vi "CreateProjectsForEachLibrary.vi"() -> ()   [LabVIEW 2019, in "DepsWatchToolsMenu.lvlib"]
uses:
  DepsWatchToolsMenu.lvlib
  vi.lib/DepsWatch/DepsWatch.lvlib
  <userlib>/_OpenG.lib/file/file.llb/Append Path to Root if Relative - Scalar__ogtk.vi
  <userlib>/_OpenG.lib/file/file.llb/Compare Two Paths - Scalar__ogtk.vi
panel:
  out "Projects Created":path[](array[path])
  out "error out":errorcluster
  in  "Build Specs Folder Path":path=path "C:/sw-deps-monitor/Source/BuildSpecs"
  in  "error in (no error)":errorcluster
  in  "Source Folder Path":path=path "C:/sw-deps-monitor/Source"
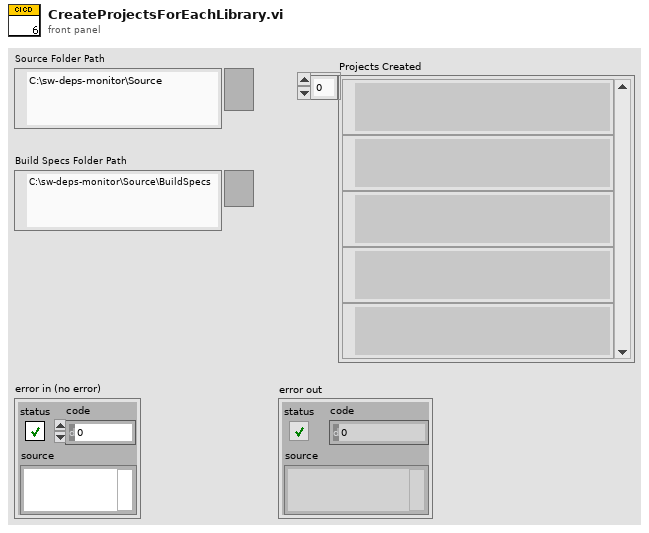
[diagram p1: front panel]
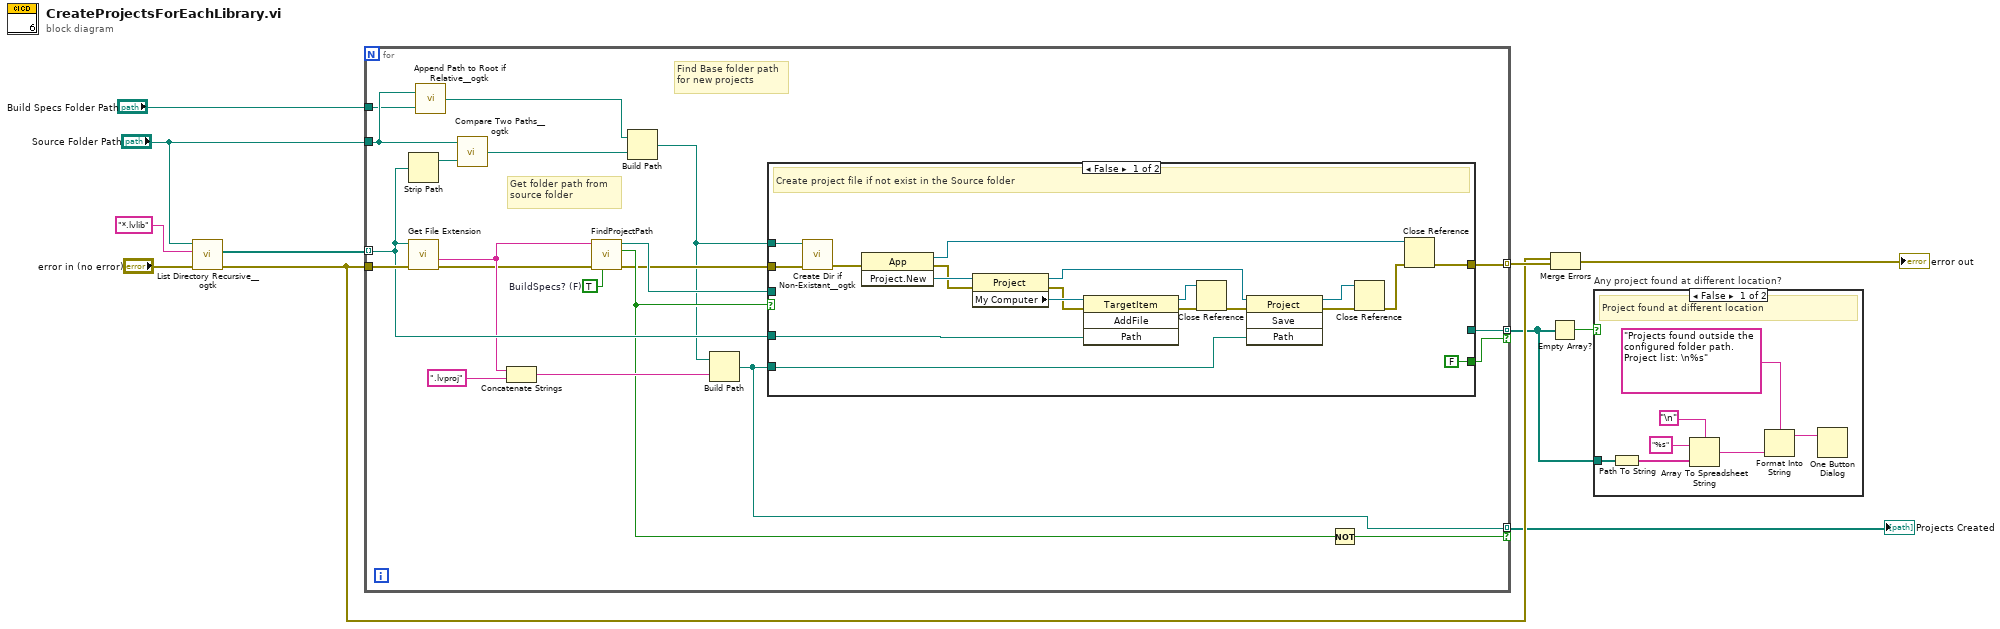
[diagram p0: block diagram]
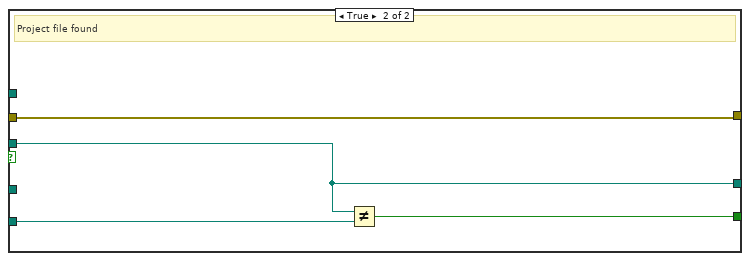
[diagram p3: hidden frame]
diagram:
  n1 = call <userlib>:"List Directory Recursive__ogtk.vi"("error in (no error)"="error in (no error)", "pattern"="*.lvlib", "Path"="Source Folder Path") -> ("error out"=w6:errorcluster, "file paths"=w9:path[])  [unwired: 5 in, 2 out]
  n2 = for {
    tunnel: w6 -> [w32]
    tunnel: w9 -> [w28] mode=indexing
    tunnel: "Build Specs Folder Path" -> [w12]
    tunnel: [w29] -> w7 mode=indexing
    tunnel: [w27] -> w4 mode=indexing if=w26
    tunnel: "Source Folder Path" -> [w13]
    tunnel: [w20] -> w1 mode=indexing if=w19
    w23 = TRUE  # BuildSpecs? (F)
    # "Find Base folder path for new projects"
    # "Get folder path from source folder"
    n3 = Strip Path(path=w28) -> (stripped path=w15:path)  [unwired: 1 out]
    n4 = call <vilib>:"Get File Extension.vi"("error in (no error)"=w32, "file"=w28) -> ("error out"=w24:errorcluster, "filename without extension"=w25:string)  [unwired: 5 in, 3 out]
    n5 = call-poly <userlib>:"Append Path to Root if Relative__ogtk.vi"("Absolute or Relative Path"=w12, "Root Path"=w13) -> ("Absolute or Appended Path"=w14:path)
    n6 = call-poly <userlib>:"Compare Two Paths__ogtk.vi"("path2"=w15, "path1"=w13) -> ("relative path from 1 to 2"=w16:path)  [unwired: 1 in, 2 out]
    n7 = Concatenate Strings(w25, ".lvproj" ("string")) -> (w30:string)
    n8 = call "FindProjectPath.vi"("BuildSpecs? (F)"=w23, "error in (no error)"=w24, "Library Name"=w25) -> ("error out"=w18:errorcluster, "Found?"=w22:bool, "Project Path"=w21:path)  [unwired: 6 in]
    n9 = Build Path(base path=w14, name or relative path=w16) -> (appended path=w17:path)
    n10 = Build Path(base path=w17, name or relative path=w30) -> (appended path=w27:path)
    n11 = case shown="False" w22 {
      tunnel: [w51 w55] -> w29
      tunnel: w28 -> [w50 _]
      tunnel: w18 -> [w35 w55]
      tunnel: w27 -> [w37 w54]
      tunnel: w21 -> [_ w53]
      tunnel: [_ w53] -> w20
      tunnel: [FALSE w52] -> w19
      tunnel: w17 -> [w34 _]
      frame False {
        # "Create project file if not exist in the Source folder"
        n12 = call <userlib>:"Create Dir if Non-Existant__ogtk.vi"("error in (no error)"=w35, "Directory Path"=w34) -> ("error out"=w33:errorcluster)  [unwired: 7 in, 2 out]
        n13 = invoke class="App" method="Project.New"(error in=w33) -> (reference out=w48:refnum<vi>, error out=w47:errorcluster, "Project:New"=w49:refnum<vi>)  [unwired: 2 in]
        n14 = property class="Project"(reference=w49, error in=w47) -> (reference out=w40:refnum<vi>, error out=w45:errorcluster, "My Computer"=w46:refnum<vi>)
        n15 = invoke class="TargetItem" method="AddFile"(reference=w46, error in=w45, "Path"=w50) -> (reference out=w44:refnum<vi>, error out=w43:errorcluster)  [unwired: 1 in, 2 out]
        n16 = Close Reference(reference=w44, error in (no error)=w43) -> (error out=w41:errorcluster)
        n17 = invoke class="Project" method="Save"(reference=w40, error in=w41, "Path"=w37) -> (reference out=w39:refnum<vi>, error out=w38:errorcluster)  [unwired: 1 in, 2 out]
        n18 = Close Reference(reference=w39, error in (no error)=w38) -> (error out=w42:errorcluster)
        n19 = Close Reference(reference=w48, error in (no error)=w42) -> (error out=w51:errorcluster)
      }
      frame True {
        # "Project file found"
        n20 = Not Equal?(x=w53, y=w54) -> (x != y?=w52:bool)
      }
    }
    n21 = Not(x=w22) -> (.not. x?=w26:bool)
  }
  "Projects Created" <- w4
  n22 = Empty Array?(array=w1) -> (empty?=w2:bool)
  n23 = Merge Errors(w6, w7) -> (→"error out":errorcluster)
  n24 = case "Any project found at different location?" shown="False" w2 {
    tunnel: w1 -> [w62 _]
    frame False {
      # "Project found at different location"
      n25 = Path To String(path=w62) -> (string=w59:string[])
      n26 = Array To Spreadsheet String(delimiter (Tab)="\n", array=w59, 3:"%s" ("format string")) -> (spreadsheet string=w58:string)
      n27 = Format Into String(format string="Projects found outside the configured folder path. Project list: \n%s", w58) -> (resulting string=w57:string)  [unwired: 2 in, 1 out]
      n28 = One Button Dialog(message=w57) -> ()  [unwired: 1 in, 1 out]
    }
    frame True {
    }
  }
